vi "Orca Flash Engine.vi"(0 "Notifier Name":string, 11 "Camera ID":string[](array[string])) -> ()   [LabVIEW 2025]
uses:
  Orca Flash Controls/Orca Flash Parameters.ctl
  Orca Flash Controls/Orca Flash Parameter List.ctl
  Orca Flash Controls/Orca Flash ROI.ctl
  Orca Flash Controls/Orca Flash Notifier Element.ctl
  Orca Flash Controls/Orca Flash Actions.ctl
  <vilib>/vision/Image Controls.llb/IMAQ Image.ctl
  Camera Controls/Camera IMAQ Key Info.ctl
panel:
  out "Last Error":errorcluster
  in  "Ext Options":cluster{"Polarity":i32, "Delay":dbl}={"Polarity"=1, "Delay"=0.0} {"Polarity" items=["Negative"=1, "Positive"=2]}
  in  "Trigger Source":i32(ring)=1 items=["Internal"=1, "External"=2, "Software"=3, "Master Pulse"=4]
  in  "Port":i32=1
  in  "Options":cluster{"Width":dbl, "Delay":dbl, "Source":u32}={"Width"=0.003, "Delay"=0.0, "Source"=2} {"Source" items=["Exposure"=1, "Readout End"=2, "V Sync"=3, "H Sync"=4, "Trigger"=6]}
  in  "Trigger Type":cluster{"Mode":u32, "Polarity":u32}={"Mode"=1, "Polarity"=2} {"Mode" items=["Low"=1, "Global Exposure"=2, "Programmable"=3, "Trigger Ready"=4, "High"=5]; "Polarity" items=["Negative"=1, "Positive"=2]}
  in  "Orca Flash ROI":T1
  in  "Use Display Module":bool
  in  "Sensor Mode":enum32{"Area", "Progressive"}(radio)
  in  "Number of lines":dbl=8.0
  in  "Internal Line Interval Setpoint":dbl=0.001
  in  "Get Parameter":bool
  in  "Set Parameter":bool
  in  "Get ROI":bool
  in  "Set ROI":bool
  in  "sCMOS Parameter":T2={"Value"=0.0, "Parameter"=2049184} {"Parameter" items=["SENSOR MODE"=4212128, "READOUT SPEED"=4211872, "READOUT DIRECTION"=4211904, "TRIGGER GLOBAL EXPOSURE"=2049680, "TRIGGER DELAY"=1066480, "SYNC READOUT SYSTEM BLANK"=1066528, "SENSOR COOLER"=2115248, "SENSOR COOLER STATUS"=2115280, "EXPOSURE TIME"=2049184, "DEFECT CORRECT MODE"=4670368, "BINNING"=4215968, "INTERNAL LINE SPEED"=4226000, "INTERNAL LINE INTERVAL"=4226016, "IMAGE PIXEL TYPE"=4343296, "NUMBER OF OUTPUT TRIGGER CONNECTOR"=1852320, "OUTPUT TRIGGER SOURCE[0]"=1852576, "OUTPUT TRIGGER SOURCE[1]"=1852832, "OUTPUT TRIGGER SOURCE[2]"=1853088, "OUTPUT TRIGGER POLARITY[0]"=1852592, "OUTPUT TRIGGER POLARITY[1]"=1852848, "OUTPUT TRIGGER POLARITY[2]"=1853104, "OUTPUT TRIGGER ACTIVE[0]"=1852608, "OUTPUT TRIGGER ACTIVE[1]"=1852864, "OUTPUT TRIGGER ACTIVE[2]"=1853120, "OUTPUT TRIGGER DELAY[0]"=1852624, "OUTPUT TRIGGER DELAY[1]"=1852880, "OUTPUT TRIGGER DELAY[2]"=1853136, "OUTPUT TRIGGER PERIOD[0]"=1852640, "OUTPUT TRIGGER PERIOD[1]"=1852896, "OUTPUT TRIGGER PERIOD[2]"=1853152, "OUTPUT TRIGGER KIND[0]"=1852656, "OUTPUT TRIGGER KIND[1]"=1852912, "OUTPUT TRIGGER KIND[2]"=1853168, "OUTPUT TRIGGER PRE HSYNC COUNT"=1852704]}
  in  "# of frames":u32=100
  in  "Path":path
  in  "Record":bool
  in  "Preview":bool
  out "Acquisition Loop":i32
  in  "QUIT":bool
  out "Acquisition Frame":i32
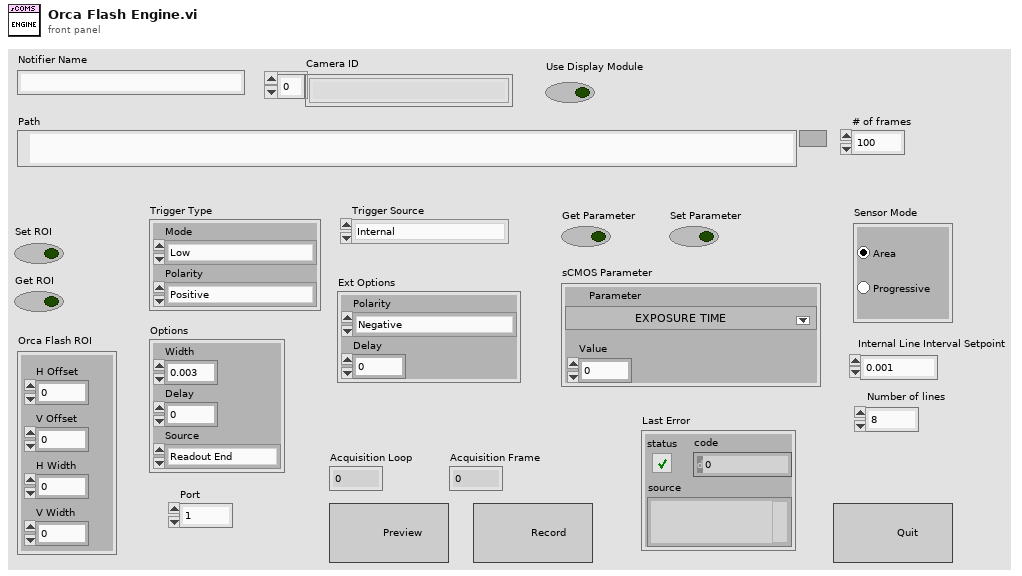
[diagram p1: front panel]
types:
  T1 = typedef "Orca Flash ROI.ctl" = cluster{"H Offset":i32, "V Offset":i32, "H Width":i32, "V Width":i32}
  T2 = typedef "Orca Flash Parameters.ctl" = cluster{"Value":dbl, "Parameter":T3}
  T3 = typedef "Orca Flash Parameter List.ctl" = u32
  T4 = typedef "Camera IMAQ Key Info.ctl" = cluster{"Frame":u32, "Sensor Height":i32, "Sensor Width":i32, "ROI Height":i32, "ROI Width":i32, "ROI Enable?":bool, "Bit per Pixel":u8}
  T5 = typedef "Image Type" = u32
  T6 = typedef "Orca Flash Notifier Element.ctl" = cluster{"Camera Actions":T7, "Received?":bool, "Running?":bool, "sCMOS Parameter":T2, "sCMOS ROI":T1, "Save Path":path, "# of frames":u32, "Image Ref":T8}
  T7 = typedef "Orca Flash Actions.ctl" = enum16{"Idle", "Preview", "Record", "Record Settings", "Set Param", "Get Param", "Set ROI", "Get ROI", "Trigger Source", "Trigger Type", "Progessive Mode", "Area Mode", "Status", "Quit"}
  T8 = typedef "IMAQ Image.ctl" = refnum<image>
  T9 = enum32{"Invalid", "Standard", "Closed", "Hidden", "Minimized", "Maximized"}
  T10 = cluster{"Horizontal Offset":i32, "Vertical Offset":i32, "Horizontal Size":i32, "Vertical Size":i32}
  T11 = typedef "LVMinMaxIncTypeDef.ctl" = cluster{"Minimum":dbl, "Maximum":dbl, "Increment":dbl}
  T12 = cluster{"H Offset":cluster{"Value":i32, "Limits":T11}, "V Offset":cluster{"Value":i32, "Limits":T11}, "H Size":cluster{"Value":i32, "Limits":T11}, "V Size":cluster{"Value":i32, "Limits":T11}}
  T13 = cluster{"Input Trigger Mode":u32, "Input Trigger Polarity":u32, "Times":u32, "Delay":dbl}
  T14 = cluster{"Output Trigger Period":dbl, "Delay":dbl, "Source":u32}
  T15 = cluster{"Output Trigger Mode":u32, "Output Trigger Polarity":u32}
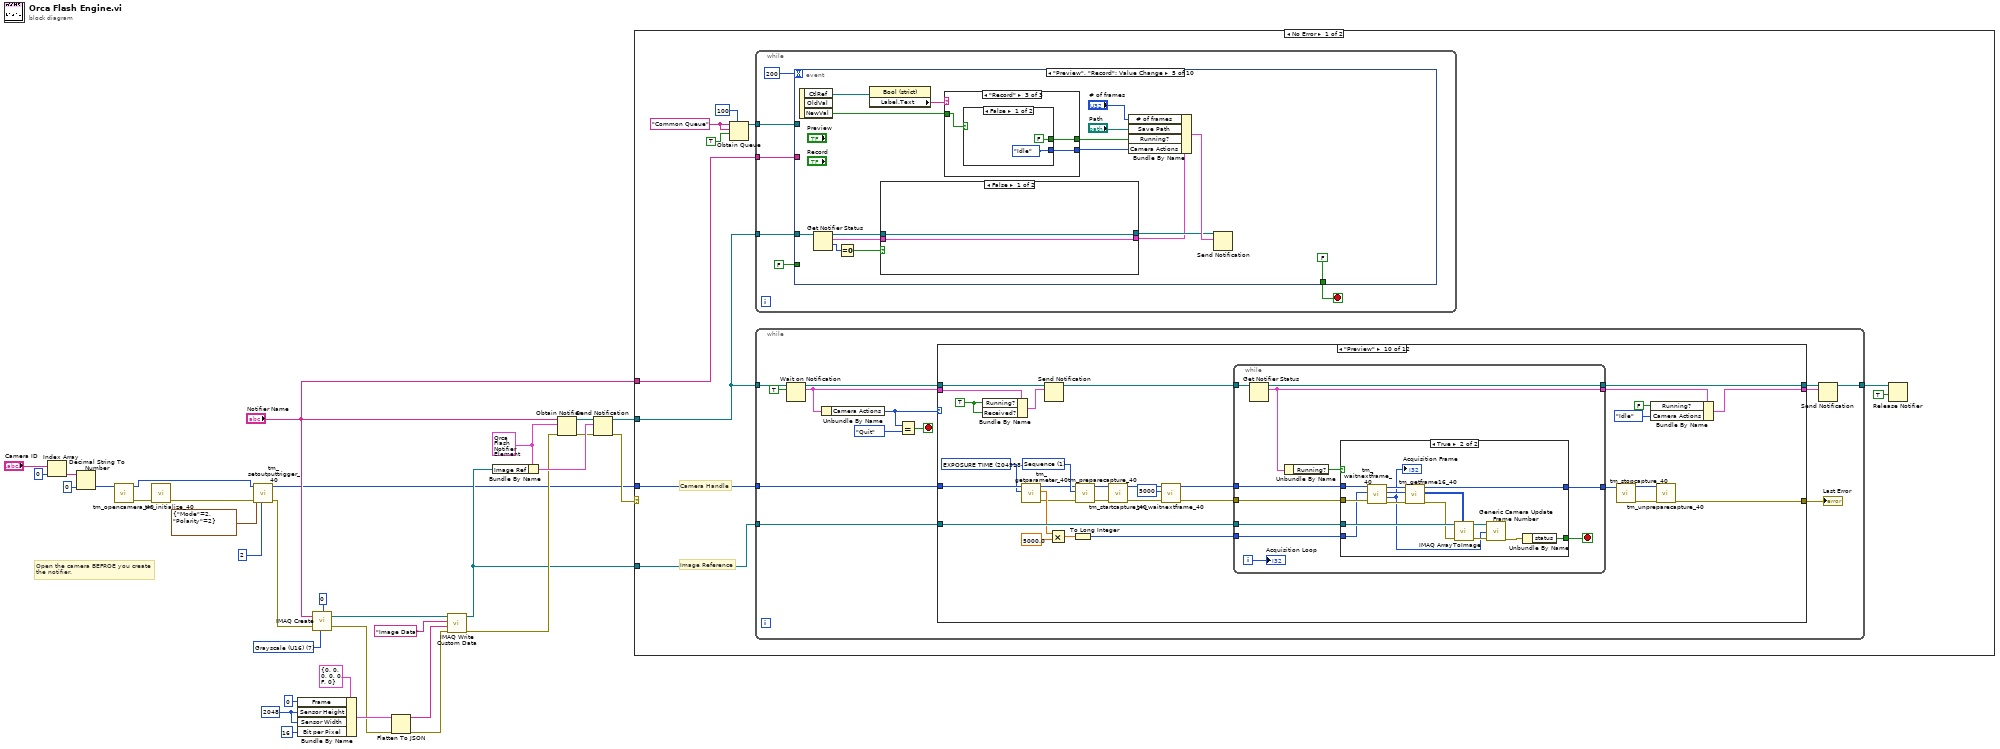
[diagram p0: block diagram]
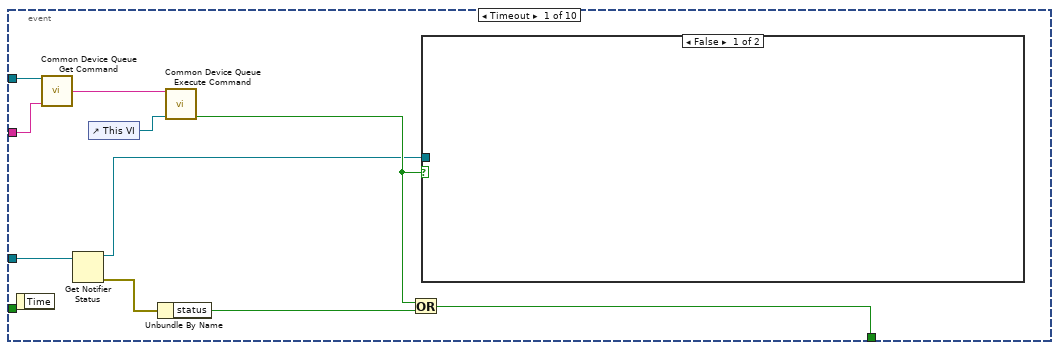
[diagram p2: hidden frame]
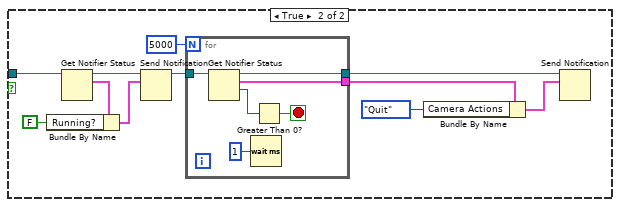
[diagram p3: hidden frame]
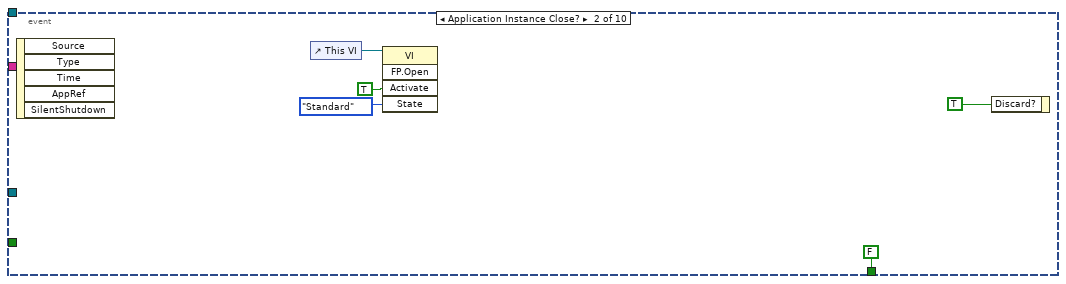
[diagram p4: hidden frame]
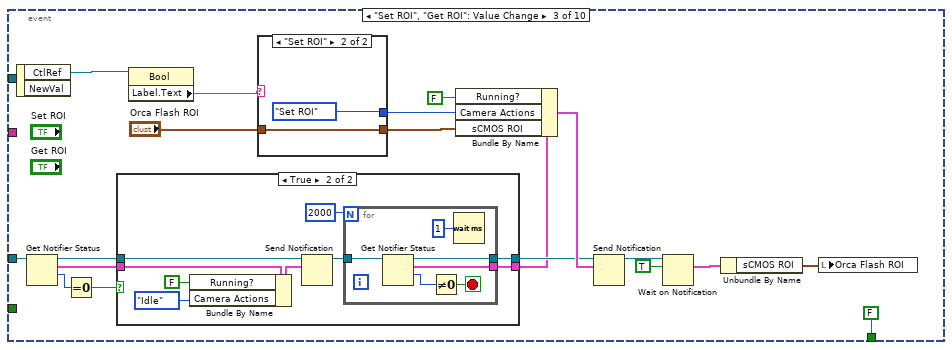
[diagram p5: hidden frame]
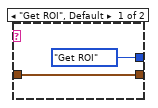
[diagram p7: hidden frame]
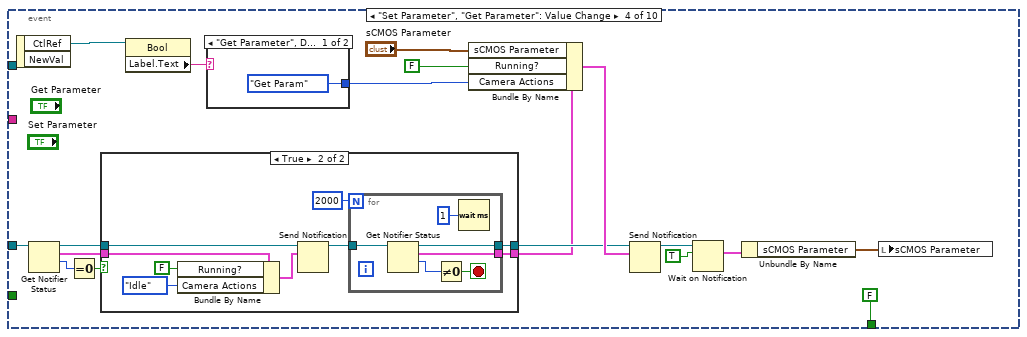
[diagram p8: hidden frame]
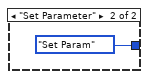
[diagram p10: hidden frame]
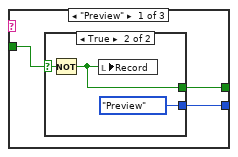
[diagram p11: hidden frame]
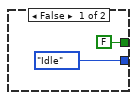
[diagram p12: hidden frame]
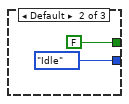
[diagram p13: hidden frame]
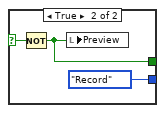
[diagram p14: hidden frame]
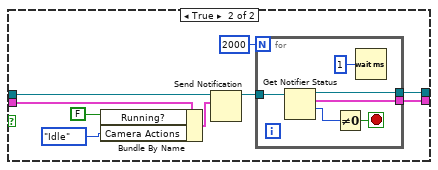
[diagram p15: hidden frame]
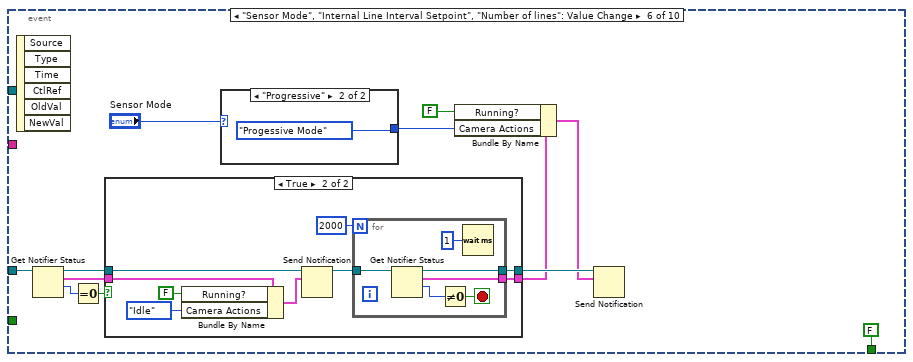
[diagram p16: hidden frame]
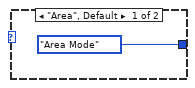
[diagram p17: hidden frame]
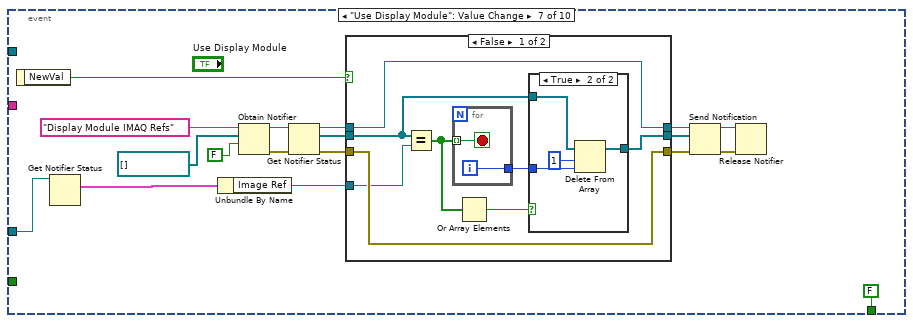
[diagram p19: hidden frame]
diagram:
  w18 = 2048 ("Sensor Height")
  w14 = T5 7 items=["Grayscale (U8)", "Grayscale (I16)", "Grayscale (SGL)", "Complex (CSG)", "RGB (U32)", "HSL (U32)", "RGB (U64)", "Grayscale (U16)"] ("Image Type")
  w28 = T6 {"Camera Actions"=enum."Idle", "Received?"=FALSE, "Running?"=FALSE, "sCMOS Parameter"={"Value"=0.0, "Parameter"=0}, "sCMOS ROI"={"H Offset"=0, "V Offset"=0, "H Width"=0, "V Width"=0}, "Save Path"=path "", "# of frames"=1, "Image Ref"=refnum} ("Camera Cluster")
  # "Open the camera BEFROE you create\nthe notifier."
  n1 = Index Array(array="Camera ID", index=0) -> (element=w31:string)
  n2 = Decimal String To Number(string=w31, default (0L)=u32 0 ("default (0 I32)")) -> (number=w24:u32)  [unwired: 1 in, 1 out]
  n3 = call <userlib>:"tm_initialize_40.vi"() -> ("error out"=w25:errorcluster)  [unwired: 8 in, 3 out]
  n4 = call <userlib>:"tm_opencamera_40.vi"("error in (no error)"=w25, "Camera Index"=w24) -> ("error out"=w4:errorcluster, "Handle out"=w3:u32)  [unwired: 7 in, 1 out]
  n5 = call <userlib>:"tm_setoutputtrigger_40.vi"("Port"=2, "error in (no error)"=w4, "Type"=cluster{"Mode":u32, "Polarity":u32} {"Mode"=2, "Polarity"=2}, "Handle in"=w3) -> ("error out"=w6:errorcluster, "Handle out"=w5:u32)  [unwired: 6 in]
  n6 = Bundle By Name(cluster=T4 {"Frame"=0, "Sensor Height"=0, "Sensor Width"=0, "ROI Height"=0, "ROI Width"=0, "ROI Enable?"=FALSE, "Bit per Pixel"=0} ("Camera IMAQ Key Info"), "Frame"=u32 0, "Sensor Height"=w18, "Sensor Width"=w18, "Bit per Pixel"=u8 16) -> (w21:T4)
  n7 = call "IMAQ Create"("Border Size"=0, "Image Name"="Notifier Name", "Image Type"=w14, "error in (no error)"=w6) -> ("New Image"=w16:T8, "error out"=w13:errorcluster)  [unwired: 1 in]
  n8 = Flatten To JSON(anything=w21, error in (no error)=w13) -> (JSON string=w22:string, 11:w12:errorcluster)  [unwired: 1 in]
  n9 = call "IMAQ Write Custom Data"("error in (no error)"=w12, "Custom Data In"=w22, "Key"="Image Data", "Image"=w16) -> ("error out"=w11:errorcluster, "Image Out"=w8:T8)  [unwired: 6 in]
  n10 = Bundle By Name(cluster=w28, "Image Ref"=w8) -> (w29:T6)
  n11 = Obtain Notifier(name (unnamed)="Notifier Name", notification data type=w28, error in (no error)=w11) -> (notifier out=w27:refnum<notifier>, error out=w26:errorcluster)  [unwired: 1 in, 1 out]
  n12 = Send Notification(notification=w29, notifier=w27, error in (no error)=w26) -> (notifier out=w10:refnum<notifier>, error out=w7:errorcluster)
  n13 = case shown="No Error" w7 {
    selector: w7 -> [_ w719]
    tunnel: w10 -> [w37 w712]
    tunnel: "Notifier Name" -> [w34 w709]
    tunnel: w8 -> [w39 _]
    tunnel: w5 -> [w38 _]
    frame No Error {
      w43 = "Common Queue" ("Unique Notifier Name")
      # "Image Reference"
      # "Camera Handle"
      n14 = Obtain Queue(max queue size (-1, unlimited)=100, name (unnamed)=w43, element data type=w43, create if not found? (T)=TRUE) -> (queue out=w40:refnum<queue>)  [unwired: 1 in, 2 out]
      n15 = while {
        tunnel: w37 -> [w47]
        tunnel: w40 -> [w46]
        tunnel: w34 -> [w45]
        stop <- w49 stop-if-true
        n16 = event shown="[4] \"Preview\", \"Record\": Value Change" {
          selector: _ -> [_ _ _ _ _ _ _ _ _ _]
          dyn-events: _ -> [_ _ _ _ _ _ _ _ _ _]
          timeout: 200 -> [_ _ _ _ _ _ _ _ _ _]
          tunnel: w47 -> [w59 _ w88 w126 w169 w217 w241 w280 w308 w341]
          tunnel: [w56 FALSE ("NewVal") FALSE ("NewVal") FALSE ("NewVal") FALSE ("NewVal") FALSE ("NewVal") FALSE ("NewVal") w289 w317 w345] -> w49
          tunnel: w46 -> [w53 _ _ _ _ _ _ _ _ _]
          tunnel: w45 -> [w52 _ _ _ _ _ _ _ _ _]
          tunnel: FALSE -> [_ _ _ _ _ _ _ w289 w317 _]
          event Timeout {
            n17 = event-data() -> ()  [unwired: 1 in, 1 out]
            n18 = call "Common Device Queue Get Command.vi"("Common Queue"=w53, "Notifier Name"=w52) -> ("Command"=w55:string)  [unwired: 12 in, 1 out]
            n19 = Get Notifier Status(notifier=w59) -> (notifier out=w50:refnum<notifier>, error out=w58:errorcluster)  [unwired: 1 in, 3 out]
            n20 = control-ref of="This VI"() -> (w54:refnum<vi>)
            n21 = Unbundle By Name(w58) -> ("status"=w57:bool)
            n22 = call "Common Device Queue Execute Command.vi"("Common Command"=w55, "VI Refnum"=w54) -> ("Quit?"=w51:bool)  [unwired: 12 in, 1 out]
            n23 = Or(x=w51, y=w57) -> (x .or. y?=w56:bool)
            n24 = case shown="False" w51 {
              tunnel: w50 -> [_ w70]
              frame False {
              }
              frame True {
                n25 = Get Notifier Status(notifier=w70) -> (notifier out=w67:refnum<notifier>, current notification=w69:T6)  [unwired: 1 in, 3 out]
                n26 = Bundle By Name(cluster=w69, "Running?"=FALSE) -> (w66:T6)
                n27 = Send Notification(notification=w66, notifier=w67) -> (notifier out=w64:refnum<notifier>)  [unwired: 1 in, 1 out]
                n28 = for {
                  N: 5000 -> [_]
                  tunnel: w64 -> [w75]
                  tunnel: [w73] -> w63
                  tunnel: [w71] -> w62
                  stop <- w74 stop-if-true
                  n29 = Get Notifier Status(notifier=w75) -> (notifier out=w73:refnum<notifier>, current notification=w71:T6, # waiting=w76:i32)  [unwired: 1 in, 2 out]
                  n30 = Wait (ms)(milliseconds to wait=u32 1) -> ()  [unwired: 1 out]
                  n31 = Greater Than 0?(x=w76) -> (x > 0?=w74:bool)
                }
                n32 = Bundle By Name(cluster=w62, "Camera Actions"=Orca_Flash_Actions."Quit") -> (w60:T6)
                n33 = Send Notification(notification=w60, notifier=w63) -> ()  [unwired: 1 in, 2 out]
              }
            }
          }
          event Application Instance Close? {
            n34 = event-data() -> ()  [unwired: 1 in, 5 out]
            n35 = control-ref of="This VI"() -> (w79:refnum<vi>)
            n36 = invoke class="VI" method="FP.Open"(reference=w79, "Activate"=TRUE ("Activate?"), "State"=T9."Standard") -> ()  [unwired: 2 in, 5 out]
            n37 = event-data("Discard?"=TRUE) -> ()  [unwired: 1 in, 1 out]
          }
          event "Set ROI", "Get ROI": Value Change {
            n38 = event-data() -> ("CtlRef"=w98:refnum<vi>)  [unwired: 1 in, 1 out]
            n39 = Get Notifier Status(notifier=w88) -> (notifier out=w86:refnum<notifier>, current notification=w85:T6, # waiting=w84:i32)  [unwired: 1 in, 2 out]
            n40 = Equal To 0?(x=w84) -> (x = 0?=w87:bool)
            n41 = case shown="True" w87 {
              tunnel: [w102 w108] -> w90
              tunnel: [w101 w107] -> w89
              tunnel: w86 -> [w102 w106]
              tunnel: w85 -> [w101 w103]
              frame False {
              }
              frame True {
                n42 = Bundle By Name(cluster=w103, "Running?"=FALSE, "Camera Actions"=Orca_Flash_Actions."Idle") -> (w110:T6)
                n43 = Send Notification(notification=w110, notifier=w106) -> (notifier out=w111:refnum<notifier>)  [unwired: 1 in, 1 out]
                n44 = for {
                  N: 2000 -> [_]
                  tunnel: w111 -> [w117]
                  tunnel: [w114] -> w108
                  tunnel: [w113] -> w107
                  stop <- w115 stop-if-true
                  n45 = Get Notifier Status(notifier=w117) -> (notifier out=w114:refnum<notifier>, current notification=w113:T6, # waiting=w116:i32)  [unwired: 1 in, 2 out]
                  n46 = Not Equal To 0?(x=w116) -> (x != 0?=w115:bool)
                  n47 = Wait (ms)(milliseconds to wait=u32 1) -> ()  [unwired: 1 out]
                }
              }
            }
            n48 = property class="Bool"(reference=w98) -> ("Label.Text"=w97:string)  [unwired: 1 in, 2 out]
            n49 = case shown="\"Set ROI\"" w97 {
              tunnel: [Orca_Flash_Actions."Get ROI" ("Camera Actions") Orca_Flash_Actions."Set ROI" ("Camera Actions")] -> w96
              tunnel: [w118 w120] -> w95
              tunnel: "Orca Flash ROI" -> [w118 w120]
              frame "Get ROI", Default {
              }
              frame "Set ROI" {
              }
            }
            n50 = Bundle By Name(cluster=w89, "Running?"=FALSE, "Camera Actions"=w96, "sCMOS ROI"=w95) -> (w94:T6)
            n51 = Send Notification(notification=w94, notifier=w90) -> (notifier out=w93:refnum<notifier>)  [unwired: 1 in, 1 out]
            n52 = Wait on Notification(notifier=w93, ignore previous (F)=TRUE) -> (notification=w92:T6)  [unwired: 2 in, 3 out]
            n53 = Unbundle By Name(w92) -> ("sCMOS ROI"=w82:T1)
            n54 = local write "Orca Flash ROI"(w82) -> ()
          }
          event "Set Parameter", "Get Parameter": Value Change {
            n55 = event-data() -> ("CtlRef"=w137:refnum<vi>)  [unwired: 1 in, 1 out]
            n56 = Get Notifier Status(notifier=w126) -> (notifier out=w124:refnum<notifier>, current notification=w123:T6, # waiting=w122:i32)  [unwired: 1 in, 2 out]
            n57 = Equal To 0?(x=w122) -> (x = 0?=w125:bool)
            n58 = case shown="True" w125 {
              tunnel: w124 -> [w141 w150]
              tunnel: w123 -> [w140 w149]
              tunnel: [w141 w145] -> w129
              tunnel: [w140 w144] -> w128
              frame False {
              }
              frame True {
                n59 = Bundle By Name(cluster=w149, "Running?"=FALSE, "Camera Actions"=Orca_Flash_Actions."Idle") -> (w147:T6)
                n60 = Send Notification(notification=w147, notifier=w150) -> (notifier out=w146:refnum<notifier>)  [unwired: 1 in, 1 out]
                n61 = for {
                  N: 2000 -> [_]
                  tunnel: w146 -> [w156]
                  tunnel: [w153] -> w145
                  tunnel: [w152] -> w144
                  stop <- w154 stop-if-true
                  n62 = Get Notifier Status(notifier=w156) -> (notifier out=w153:refnum<notifier>, current notification=w152:T6, # waiting=w155:i32)  [unwired: 1 in, 2 out]
                  n63 = Not Equal To 0?(x=w155) -> (x != 0?=w154:bool)
                  n64 = Wait (ms)(milliseconds to wait=u32 1) -> ()  [unwired: 1 out]
                }
              }
            }
            n65 = property class="Bool"(reference=w137) -> ("Label.Text"=w136:string)  [unwired: 1 in, 2 out]
            n66 = case shown="\"Get Parameter\", Default" w136 {
              tunnel: [Orca_Flash_Actions."Get Param" ("Camera Actions") Orca_Flash_Actions."Set Param" ("Camera Actions")] -> w135
              frame "Get Parameter", Default {
              }
              frame "Set Parameter" {
              }
            }
            n67 = Bundle By Name(cluster=w128, "sCMOS Parameter"="sCMOS Parameter", "Running?"=FALSE, "Camera Actions"=w135) -> (w134:T6)
            n68 = Send Notification(notification=w134, notifier=w129) -> (notifier out=w133:refnum<notifier>)  [unwired: 1 in, 1 out]
            n69 = Wait on Notification(notifier=w133, ignore previous (F)=TRUE) -> (notification=w132:T6)  [unwired: 2 in, 3 out]
            n70 = Unbundle By Name(w132) -> ("sCMOS Parameter"=w131:T2)
            n71 = local write "sCMOS Parameter"(w131) -> ()
          }
          event "Preview", "Record": Value Change {
            n72 = event-data() -> ("CtlRef"=w173:refnum<vi>, "NewVal"=w171:bool)  [unwired: 1 in, 1 out]
            n73 = Get Notifier Status(notifier=w169) -> (notifier out=w161:refnum<notifier>, current notification=w160:T6, # waiting=w159:i32)  [unwired: 1 in, 2 out]
            n74 = Equal To 0?(x=w159) -> (x = 0?=w162:bool)
            n75 = property class="Bool (strict)"(reference=w173) -> ("Label.Text"=w172:string)  [unwired: 1 in, 2 out]
            n76 = case shown="False" w162 {
              tunnel: w161 -> [w194 w203]
              tunnel: [w194 w199] -> w164
              tunnel: [w193 w197] -> w163
              tunnel: w160 -> [w193 w196]
              frame False {
              }
              frame True {
                n77 = Bundle By Name(cluster=w196, "Running?"=FALSE, "Camera Actions"=Orca_Flash_Actions."Idle") -> (w201:T6)
                n78 = Send Notification(notification=w201, notifier=w203) -> (notifier out=w200:refnum<notifier>)  [unwired: 1 in, 1 out]
                n79 = for {
                  N: 2000 -> [_]
                  tunnel: w200 -> [w209]
                  tunnel: [w208] -> w199
                  tunnel: [w207] -> w197
                  stop <- w205 stop-if-true
                  n80 = Get Notifier Status(notifier=w209) -> (notifier out=w208:refnum<notifier>, current notification=w207:T6, # waiting=w206:i32)  [unwired: 1 in, 2 out]
                  n81 = Not Equal To 0?(x=w206) -> (x != 0?=w205:bool)
                  n82 = Wait (ms)(milliseconds to wait=u32 1) -> ()  [unwired: 1 out]
                }
              }
            }
            n83 = case shown="\"Record\"" w172 {
              tunnel: w171 -> [w177 _ w187]
              tunnel: [w176 FALSE w186] -> w167
              tunnel: [w175 Orca_Flash_Actions."Idle" ("Camera Actions") w185] -> w170
              frame "Preview" {
                n84 = case shown="True" w177 {
                  selector: w177 -> [_ w182]
                  tunnel: [FALSE w181] -> w176
                  tunnel: [Orca_Flash_Actions."Idle" ("Camera Actions") Orca_Flash_Actions."Preview" ("Camera Actions")] -> w175
                  frame False {
                  }
                  frame True {
                    n85 = Not(x=w182) -> (.not. x?=w181:bool)
                    n86 = local write "Record"(w181) -> ()
                  }
                }
              }
              frame Default {
              }
              frame "Record" {
                n87 = case shown="False" w187 {
                  selector: w187 -> [_ w192]
                  tunnel: [FALSE w191] -> w186
                  tunnel: [Orca_Flash_Actions."Idle" ("Camera Actions") Orca_Flash_Actions."Record" ("Camera Actions")] -> w185
                  frame False {
                  }
                  frame True {
                    n88 = Not(x=w192) -> (.not. x?=w191:bool)
                    n89 = local write "Preview"(w191) -> ()
                  }
                }
              }
            }
            n90 = Bundle By Name(cluster=w163, "# of frames"="# of frames", "Save Path"="Path", "Running?"=w167, "Camera Actions"=w170) -> (w168:T6)
            n91 = Send Notification(notification=w168, notifier=w164) -> ()  [unwired: 1 in, 2 out]
          }
          event "Sensor Mode", "Internal Line Interval Setpoint", "Number of lines": Value Change {
            n92 = event-data() -> ()  [unwired: 1 in, 6 out]
            n93 = Get Notifier Status(notifier=w217) -> (notifier out=w220:refnum<notifier>, current notification=w219:T6, # waiting=w218:i32)  [unwired: 1 in, 2 out]
            n94 = Equal To 0?(x=w218) -> (x = 0?=w221:bool)
            n95 = case shown="True" w221 {
              tunnel: w220 -> [w225 w234]
              tunnel: w219 -> [w224 w233]
              tunnel: [w225 w229] -> w216
              tunnel: [w224 w228] -> w215
              frame False {
              }
              frame True {
                n96 = Bundle By Name(cluster=w233, "Running?"=FALSE, "Camera Actions"=Orca_Flash_Actions."Idle") -> (w231:T6)
                n97 = Send Notification(notification=w231, notifier=w234) -> (notifier out=w230:refnum<notifier>)  [unwired: 1 in, 1 out]
                n98 = for {
                  N: 2000 -> [_]
                  tunnel: w230 -> [w240]
                  tunnel: [w237] -> w229
                  tunnel: [w236] -> w228
                  stop <- w238 stop-if-true
                  n99 = Get Notifier Status(notifier=w240) -> (notifier out=w237:refnum<notifier>, current notification=w236:T6, # waiting=w239:i32)  [unwired: 1 in, 2 out]
                  n100 = Not Equal To 0?(x=w239) -> (x != 0?=w238:bool)
                  n101 = Wait (ms)(milliseconds to wait=u32 1) -> ()  [unwired: 1 out]
                }
              }
            }
            n102 = case shown="\"Progressive\"" "Sensor Mode" {
              tunnel: [Orca_Flash_Actions."Area Mode" ("Camera Actions") Orca_Flash_Actions."Progessive Mode" ("Camera Actions")] -> w211
              frame "Area", Default {
              }
              frame "Progressive" {
              }
            }
            n103 = Bundle By Name(cluster=w215, "Running?"=FALSE, "Camera Actions"=w211) -> (w210:T6)
            n104 = Send Notification(notification=w210, notifier=w216) -> ()  [unwired: 1 in, 2 out]
          }
          event "Use Display Module": Value Change {
            n105 = event-data() -> ("NewVal"=w242:bool)  [unwired: 1 in]
            n106 = Get Notifier Status(notifier=w241) -> (current notification=w243:T6)  [unwired: 1 in, 4 out]
            n107 = Unbundle By Name(w243) -> ("Image Ref"=w257:T8)
            n108 = Obtain Notifier(name (unnamed)="Display Module IMAQ Refs", notification data type=T8[] [], create if not found? (T)=FALSE) -> (notifier out=w250:refnum<notifier>, error out=w251:errorcluster)  [unwired: 1 in, 1 out]
            n109 = Get Notifier Status(notifier=w250, error in (no error)=w251) -> (notifier out=w249:refnum<notifier>, current notification=w247:T8[], error out=w248:errorcluster)  [unwired: 2 out]
            n110 = case shown="False" w242 {
              tunnel: w249 -> [w266 w276]
              tunnel: w248 -> [w260 w275]
              tunnel: w247 -> [w262 w278]
              tunnel: [w261 w277] -> w244
              tunnel: [w266 w276] -> w246
              tunnel: [w260 w275] -> w245
              tunnel: w257 -> [w259 w274]
              frame False {
                n111 = Equal?(x=w262, y=w259) -> (x = y?=w265:bool[])
                n112 = for {
                  tunnel: w265 -> [w273] mode=indexing
                  tunnel: [w272] -> w263
                  i -> [w272]
                  stop <- w273 stop-if-true
                }
                n113 = Or Array Elements(Boolean array=w265) -> (logical OR=w264:bool)
                n114 = case shown="True" w264 {
                  tunnel: w263 -> [_ w270]
                  tunnel: w262 -> [w267 w269]
                  tunnel: [w267 w268] -> w261
                  frame False {
                  }
                  frame True {
                    n115 = Delete From Array(array=w269, length=1, index=w270) -> (array with subset deleted=w268:T8[])  [unwired: 1 out]
                  }
                }
              }
              frame True {
                n116 = Build Array (concatenate)(w278, w274) -> (w277:T8[])
              }
            }
            n117 = Send Notification(notification=w244, notifier=w246, error in (no error)=w245) -> (notifier out=w252:refnum<notifier>, error out=w253:errorcluster)
            n118 = Release Notifier(notifier=w252, error in (no error)=w253) -> ()  [unwired: 1 in, 3 out]
          }
          event "Trigger Type", "Options", "Port": Value Change {
            n119 = event-data() -> ()  [unwired: 1 in, 1 out]
            n120 = Get Notifier Status(notifier=w280) -> (notifier out=w287:refnum<notifier>, current notification=w286:T6, # waiting=w285:i32)  [unwired: 1 in, 2 out]
            n121 = Equal To 0?(x=w285) -> (x = 0?=w288:bool)
            n122 = case shown="True" w288 {
              tunnel: w287 -> [w291 w300]
              tunnel: w286 -> [w290 w299]
              tunnel: [w291 w295] -> w284
              tunnel: [w290 w294] -> w283
              frame False {
              }
              frame True {
                n123 = Bundle By Name(cluster=w299, "Running?"=FALSE, "Camera Actions"=Orca_Flash_Actions."Idle") -> (w297:T6)
                n124 = Send Notification(notification=w297, notifier=w300) -> (notifier out=w296:refnum<notifier>)  [unwired: 1 in, 1 out]
                n125 = for {
                  N: 2000 -> [_]
                  tunnel: w296 -> [w306]
                  tunnel: [w303] -> w295
                  tunnel: [w302] -> w294
                  stop <- w304 stop-if-true
                  n126 = Get Notifier Status(notifier=w306) -> (notifier out=w303:refnum<notifier>, current notification=w302:T6, # waiting=w305:i32)  [unwired: 1 in, 2 out]
                  n127 = Not Equal To 0?(x=w305) -> (x != 0?=w304:bool)
                  n128 = Wait (ms)(milliseconds to wait=u32 1) -> ()  [unwired: 1 out]
                }
              }
            }
            n129 = Bundle By Name(cluster=w283, "Running?"=FALSE, "Camera Actions"=Orca_Flash_Actions."Trigger Type") -> (w281:T6)
            n130 = Send Notification(notification=w281, notifier=w284) -> ()  [unwired: 1 in, 2 out]
          }
          event "Trigger Source", "Ext Options": Value Change {
            n131 = event-data() -> ()  [unwired: 1 in, 1 out]
            n132 = Get Notifier Status(notifier=w308) -> (notifier out=w315:refnum<notifier>, current notification=w314:T6, # waiting=w313:i32)  [unwired: 1 in, 2 out]
            n133 = Equal To 0?(x=w313) -> (x = 0?=w316:bool)
            n134 = case shown="True" w316 {
              tunnel: w315 -> [w319 w328]
              tunnel: w314 -> [w318 w327]
              tunnel: [w319 w323] -> w312
              tunnel: [w318 w322] -> w311
              frame False {
              }
              frame True {
                n135 = Bundle By Name(cluster=w327, "Running?"=FALSE, "Camera Actions"=Orca_Flash_Actions."Idle") -> (w325:T6)
                n136 = Send Notification(notification=w325, notifier=w328) -> (notifier out=w324:refnum<notifier>)  [unwired: 1 in, 1 out]
                n137 = for {
                  N: 2000 -> [_]
                  tunnel: w324 -> [w334]
                  tunnel: [w331] -> w323
                  tunnel: [w330] -> w322
                  stop <- w332 stop-if-true
                  n138 = Get Notifier Status(notifier=w334) -> (notifier out=w331:refnum<notifier>, current notification=w330:T6, # waiting=w333:i32)  [unwired: 1 in, 2 out]
                  n139 = Not Equal To 0?(x=w333) -> (x != 0?=w332:bool)
                  n140 = Wait (ms)(milliseconds to wait=u32 1) -> ()  [unwired: 1 out]
                }
              }
            }
            n141 = Bundle By Name(cluster=w311, "Running?"=FALSE, "Camera Actions"=Orca_Flash_Actions."Trigger Source") -> (w309:T6)
            n142 = Send Notification(notification=w309, notifier=w312) -> ()  [unwired: 1 in, 2 out]
          }
          event "QUIT": Value Change {
            n143 = event-data() -> ("NewVal"=w345:bool)  [unwired: 1 in]
            n144 = Get Notifier Status(notifier=w341) -> (notifier out=w337:refnum<notifier>, current notification=w336:T6, # waiting=w335:i32)  [unwired: 1 in, 2 out]
            n145 = Equal To 0?(x=w335) -> (x = 0?=w338:bool)
            n146 = case shown="True" w338 {
              tunnel: w337 -> [w347 w352]
              tunnel: [w347 w350] -> w340
              tunnel: [w346 w349] -> w339
              tunnel: w336 -> [w346 w348]
              frame False {
              }
              frame True {
                n147 = Bundle By Name(cluster=w348, "Running?"=FALSE, "Camera Actions"=Orca_Flash_Actions."Idle") -> (w351:T6)
                n148 = Send Notification(notification=w351, notifier=w352) -> (notifier out=w355:refnum<notifier>)  [unwired: 1 in, 1 out]
                n149 = for {
                  N: 2000 -> [_]
                  tunnel: w355 -> [w362]
                  tunnel: [w359] -> w350
                  tunnel: [w358] -> w349
                  stop <- w360 stop-if-true
                  n150 = Get Notifier Status(notifier=w362) -> (notifier out=w359:refnum<notifier>, current notification=w358:T6, # waiting=w361:i32)  [unwired: 1 in, 2 out]
                  n151 = Not Equal To 0?(x=w361) -> (x != 0?=w360:bool)
                  n152 = Wait (ms)(milliseconds to wait=u32 1) -> ()  [unwired: 1 out]
                }
              }
            }
            n153 = Bundle By Name(cluster=w339, "Running?"=FALSE, "Camera Actions"=Orca_Flash_Actions."Quit") -> (w344:T6)
            n154 = Send Notification(notification=w344, notifier=w340) -> ()  [unwired: 1 in, 2 out]
          }
        }
      }
      n155 = while {
        tunnel: w37 -> [w375]
        tunnel: w39 -> [w374]
        tunnel: w38 -> [w373]
        tunnel: [w372] -> w35
        stop <- w371 stop-if-true
        n156 = Wait on Notification(notifier=w375, ignore previous (F)=TRUE) -> (notifier out=w368:refnum<notifier>, notification=w367:T6)  [unwired: 2 in, 2 out]
        n157 = Unbundle By Name(w367) -> ("Camera Actions"=w365:T7)
        n158 = Equal?(x=w365, y=Orca_Flash_Actions."Quit") -> (x = y?=w371:bool)
        n159 = case shown="\"Preview\"" w365 {
          tunnel: w373 -> [_ w386 w430 w433 w478 w487 w502 w534 w559 w581 w637 w702]
          tunnel: [errorcluster {"status"=FALSE, "code"=0, "source"=""} ("error out") w384 w429 w462 w477 w486 w501 w522 w549 w589 w649 w701] -> w363
          tunnel: w368 -> [w380 w390 w431 w469 w483 w485 w500 w548 w568 w599 w667 w708]
          tunnel: w374 -> [_ _ _ w444 _ _ _ _ _ w586 w646 w703]
          tunnel: w367 -> [w378 w382 w427 w465 w480 w484 w499 w545 w556 w594 w658 w706]
          tunnel: [w380 w390 w431 w469 w483 w485 w500 w548 w568 w595 w659 w708] -> w369
          tunnel: [w377 w389 w423 w464 w479 w484 w499 w544 w555 w590 w654 w705] -> w366
          frame "Idle", Default {
            w379 = FALSE ("Running?")
            n160 = Bundle By Name(cluster=w378, "Received?"=w379, "Running?"=w379) -> (w377:T6)
          }
          frame "Set Param" {
            n161 = Unbundle By Name(w382) -> ("sCMOS Parameter.Parameter"=w381:T3, "sCMOS Parameter.Value"=w385:dbl)
            n162 = case shown="Default" w381 {
              selector: w381 -> [w392 _]
              tunnel: w386 -> [w399 w405]
              tunnel: w385 -> [w398 w415]
              tunnel: [w396 w406] -> w384
              tunnel: [w394 0.0 ("Value out")] -> w383
              frame Default {
                w393 = u32 4212128 items=["SENSOR MODE"=4212128, "READOUT SPEED"=4211872, "READOUT DIRECTION"=4211904, "TRIGGER GLOBAL EXPOSURE"=2049680, "TRIGGER DELAY"=1066480, "INTERNAL TRIGGER HANDLING"=1066496, "SYNC READOUT SYSTEM BLANK"=1066528, "SENSOR TEMPERATURE"=2115232, "SENSOR COOLER STATUS"=2115280, "EXPOSURE TIME"=2049184, "DEFECT CORRECT MODE"=4670368, "BINNING"=4215968, "INTERNAL LINE SPEED"=4226000, "INTERNAL LINE INTERVAL"=4226016, "NUMBER OF OUTPUT TRIGGER CONNECTOR"=1852320, "OUTPUT TRIGGER SOURCE[0]"=1852576, "OUTPUT TRIGGER SOURCE[1]"=1852832, "OUTPUT TRIGGER SOURCE[2]"=1853088, "OUTPUT TRIGGER POLARITY[0]"=1852592, "OUTPUT TRIGGER POLARITY[1]"=1852848, "OUTPUT TRIGGER POLARITY[2]"=1853104, "OUTPUT TRIGGER ACTIVE[0]"=1852608, "OUTPUT TRIGGER ACTIVE[1]"=1852864, "OUTPUT TRIGGER ACTIVE[2]"=1853120, "OUTPUT TRIGGER DELAY[0]"=1852624, "OUTPUT TRIGGER DELAY[1]"=1852880, "OUTPUT TRIGGER DELAY[2]"=1853136, "OUTPUT TRIGGER PERIOD[0]"=1852640, "OUTPUT TRIGGER PERIOD[1]"=1852896, "OUTPUT TRIGGER PERIOD[2]"=1853152, "OUTPUT TRIGGER KIND[0]"=1852656, "OUTPUT TRIGGER KIND[1]"=1852912, "OUTPUT TRIGGER KIND[2]"=1853168, "OUTPUT TRIGGER BASE SENSOR[0]"=1852672, "OUTPUT TRIGGER BASE SENSOR[1]"=1852928, "OUTPUT TRIGGER BASE SENSOR[2]"=1853184, "OUTPUT TRIGGER PRE HSYNC COUNT"=1852704] ("Parameter")
                n163 = Type Cast(type=w393, x=w392) -> (*(type *) &x=w391:u32)
                n164 = call <userlib>:"tm_setparameter_40.vi"("Value in"=w398, "Parameter"=w391, "Handle in"=w399) -> ("error out"=w397:errorcluster, "Handle out"=w395:u32)  [unwired: 7 in]
                n165 = call <userlib>:"tm_getparameter_40.vi"("error in (no error)"=w397, "Parameter"=w391, "Handle in"=w395) -> ("error out"=w396:errorcluster, "Value out"=w394:dbl)  [unwired: 6 in, 1 out]
              }
              frame 0 {
                w401 = 1 items=["Internal"=1, "External"=2, "Software"=3, "Master Pulse"=4] ("Trigger Source 2")
                w403 = 2 items=["Internal"=1, "External"=2, "Software"=3, "Master Pulse"=4] ("Trigger Source 2")
                n166 = Greater Than 0?(x=w415) -> (x > 0?=w404:bool)
                n167 = Select(t=w403, s=w404, f=w401) -> (s? t:f=w402:i32)
                n168 = call <userlib>:"tm_inputtriggersource_40.vi"("External Options"=cluster{"Polarity":i32, "Delay":dbl} {"Polarity"=2, "Delay"=0.0} ("Ext Options 2"), "Source"=w402, "Handle in"=w405) -> ("error out"=w412:errorcluster, "Handle out"=w411:u32)  [unwired: 7 in]
                n169 = case shown="2" w402 {
                  tunnel: w411 -> [w417 w422]
                  tunnel: w412 -> [w416 w421]
                  tunnel: [w417 w419] -> w413
                  tunnel: [w416 w418] -> w414
                  frame Default {
                  }
                  frame 2 {
                    w420 = 1 items=["Edge"=1, "Level"=2, "Sync Readout"=3, "Point"=4] ("Active")
                    n170 = call <userlib>:"tm_inputtriggeractive_40.vi"("error in (no error)"=w421, "Active"=w420, "Handle in"=w422) -> ("error out"=w418:errorcluster, "Handle out"=w419:u32)  [unwired: 7 in]
                  }
                }
                n171 = call <userlib>:"tm_setoutputtrigger_40.vi"("Port"=0 ("Port 2"), "error in (no error)"=w414, "Programmable Options"=cluster{"Width":dbl, "Delay":dbl, "Source":u32} {"Width"=0.003, "Delay"=0.0, "Source"=2} ("Options 2"), "Type"=cluster{"Mode":u32, "Polarity":u32} {"Mode"=4, "Polarity"=2} ("Trigger Type 2"), "Handle in"=w413) -> ("error out"=w406:errorcluster)  [unwired: 5 in, 1 out]
              }
            }
            n172 = Bundle By Name(cluster=w382, "Received?"=TRUE ("Running?"), "Camera Actions"=Orca_Flash_Actions."Idle", "sCMOS Parameter.Value"=w383) -> (w389:T6)
          }
          frame "Get Param" {
            n173 = Unbundle By Name(w427) -> ("sCMOS Parameter.Parameter"=w428:T3)
            n174 = call <userlib>:"tm_getparameter_40.vi"("Parameter"=w428, "Handle in"=w430) -> ("error out"=w429:errorcluster, "Value out"=w424:dbl)  [unwired: 7 in, 1 out]
            n175 = Bundle By Name(cluster=w427, "Received?"=TRUE ("Running?"), "Camera Actions"=Orca_Flash_Actions."Idle", "sCMOS Parameter.Value"=w424) -> (w423:T6)
          }
          frame "Set ROI" {
            w451 = "Image Data" ("Key")
            n176 = Unbundle By Name(w465) -> ("sCMOS ROI.H Offset"=w441:i32, "sCMOS ROI.V Offset"=w440:i32, "sCMOS ROI.H Width"=w439:i32, "sCMOS ROI.V Width"=w438:i32)
            n177 = call "Orca Flash Fix ROI Size.vi"("Requested Value 1"=w441, "Allowed Increment"=4, "Requested Value 2"=w440, "Requested Value 3"=w439, "Requested Value 4"=w438) -> ("Resulting Value 1"=w437:i32, "Resulting Value 2"=w436:i32, "Resulting Value 3"=w435:i32, "Resulting Value 4"=w434:i32)  [unwired: 7 in]
            n178 = Bundle By Name(cluster=T10 {"Horizontal Offset"=0, "Vertical Offset"=0, "Horizontal Size"=0, "Vertical Size"=0} ("Sub Region"), "Horizontal Offset"=w437, "Vertical Offset"=w436, "Horizontal Size"=w435, "Vertical Size"=w434) -> (w455:T10)
            n179 = call <userlib>:"tm_setarea_40.vi"("Sub Region"=w455, "Handle in"=w433) -> ("error out"=w463:errorcluster, "Handle out"=w468:u32)  [unwired: 8 in]
            n180 = call <userlib>:"tm_getarea_40.vi"("error in (no error)"=w463, "Handle in"=w468) -> ("error out"=w462:errorcluster, "Sub Region"=w461:T12)  [unwired: 7 in, 1 out]
            n181 = Unbundle By Name(w461) -> ("H Offset.Value"=w459:i32, "V Offset.Value"=w458:i32, "H Size.Value"=w442:i32, "V Size.Value"=w443:i32)
            n182 = Bundle By Name(cluster=T1 {"H Offset"=0, "V Offset"=0, "H Width"=0, "V Width"=0} ("Orca Flash ROI"), "H Offset"=w459, "V Offset"=w458, "H Width"=w442, "V Width"=w443) -> (w457:T1)
            n183 = Bundle By Name(cluster=w465, "Received?"=TRUE ("Running?"), "Camera Actions"=Orca_Flash_Actions."Idle", "sCMOS ROI"=w457) -> (w464:T6)
            n184 = call "IMAQ Read Custom Data"("Key"=w451, "Image"=w444) -> ("error out"=w452:errorcluster, "Custom Data Out"=w447:string, "Image (duplicate)"=w445:T8)  [unwired: 7 in]
            n185 = Unflatten From JSON(JSON string=w447, type and defaults=T4 {"Frame"=0, "Sensor Height"=0, "Sensor Width"=0, "ROI Height"=0, "ROI Width"=0, "ROI Enable?"=FALSE, "Bit per Pixel"=0} ("Camera IMAQ Key Info"), error in (no error)=w452) -> (value=w448:T4, error out=w453:errorcluster)  [unwired: 4 in]
            n186 = Bundle By Name(cluster=w448, "ROI Width"=w442, "ROI Height"=w443) -> (w449:T4)
            n187 = Flatten To JSON(anything=w449, error in (no error)=w453) -> (JSON string=w450:string, 11:w454:errorcluster)  [unwired: 1 in]
            n188 = call "IMAQ Write Custom Data"("error in (no error)"=w454, "Custom Data In"=w450, "Key"=w451, "Image"=w445) -> ()  [unwired: 6 in, 2 out]
          }
          frame "Get ROI" {
            n189 = call <userlib>:"tm_getarea_40.vi"("Handle in"=w478) -> ("error out"=w477:errorcluster, "Sub Region"=w476:T12)  [unwired: 8 in, 1 out]
            n190 = Unbundle By Name(w476) -> ("H Offset.Value"=w471:i32, "V Offset.Value"=w472:i32, "H Size.Value"=w473:i32, "V Size.Value"=w474:i32)
            n191 = Bundle By Name(cluster=T1 {"H Offset"=0, "V Offset"=0, "H Width"=0, "V Width"=0} ("Orca Flash ROI"), "H Offset"=w471, "V Offset"=w472, "H Width"=w473, "V Width"=w474) -> (w470:T1)
            n192 = Bundle By Name(cluster=w480, "Received?"=TRUE ("Running?"), "Camera Actions"=Orca_Flash_Actions."Idle", "sCMOS ROI"=w470) -> (w479:T6)
          }
          frame "Trigger Source" {
            n193 = call <userlib>:"tm_inputtriggersource_40.vi"("External Options"="Ext Options", "Source"="Trigger Source", "Handle in"=w487) -> ("error out"=w490:errorcluster, "Handle out"=w489:u32)  [unwired: 7 in]
            n194 = case shown="2" "Trigger Source" {
              tunnel: w489 -> [w493 w498]
              tunnel: w490 -> [w492 w497]
              tunnel: [w493 w495] -> _
              tunnel: [w492 w494] -> w486
              frame Default {
              }
              frame 2 {
                w496 = 1 items=["Edge"=1, "Level"=2, "Sync Readout"=3, "Point"=4] ("Active")
                n195 = call <userlib>:"tm_inputtriggeractive_40.vi"("error in (no error)"=w497, "Active"=w496, "Handle in"=w498) -> ("error out"=w494:errorcluster, "Handle out"=w495:u32)  [unwired: 7 in]
              }
            }
          }
          frame "Trigger Type" {
            n196 = call <userlib>:"tm_setoutputtrigger_40.vi"("Port"="Port", "Programmable Options"="Options", "Type"="Trigger Type", "Handle in"=w502) -> ("error out"=w501:errorcluster)  [unwired: 6 in, 1 out]
          }
          frame "Progessive Mode" {
            w511 = u32 2 items=["Exposure"=1, "Readout End"=2, "V Sync"=3, "H Sync"=4, "Trigger"=6] ("Source")
            w513 = u32 2 items=["NEGATIVE"=1, "POSITIVE"=2] ("Output Trigger Polarity")
            w512 = u32 3 items=["LOW"=1, "GLOBAL EXPOSURE"=2, "PROGRAMMABLE"=3, "TRIGGER READY"=4, "HIGH"=5] ("Output Trigger Mode")
            w520 = u32 2 items=["NEGATIVE"=1, "POSITIVE"=2] ("Input Trigger Polarity")
            w519 = u32 1 items=["INTERNAL"=1, "EXTERNAL EDGE"=2, "EXTERNAL LEVEL"=4, "SOFTWARE"=32, "FAST REPETITION"=64, "TDI"=128, "START"=512, "SYNC READOUT"=1024] ("Input Trigger Mode")
            w521 = u32 2049184 items=["SENSOR MODE"=4212128, "READOUT SPEED"=4211872, "READOUT DIRECTION"=4211904, "TRIGGER GLOBAL EXPOSURE"=2049680, "TRIGGER DELAY"=1066480, "INTERNAL TRIGGER HANDLING"=1066496, "SYNC READOUT SYSTEM BLANK"=1066528, "SENSOR TEMPERATURE"=2115232, "SENSOR COOLER STATUS"=2115280, "EXPOSURE TIME"=2049184, "DEFECT CORRECT MODE"=4670368, "BINNING"=4215968, "INTERNAL LINE SPEED"=4226000, "INTERNAL LINE INTERVAL"=4226016, "NUMBER OF OUTPUT TRIGGER CONNECTOR"=1852320, "OUTPUT TRIGGER SOURCE[0]"=1852576, "OUTPUT TRIGGER SOURCE[1]"=1852832, "OUTPUT TRIGGER SOURCE[2]"=1853088, "OUTPUT TRIGGER POLARITY[0]"=1852592, "OUTPUT TRIGGER POLARITY[1]"=1852848, "OUTPUT TRIGGER POLARITY[2]"=1853104, "OUTPUT TRIGGER ACTIVE[0]"=1852608, "OUTPUT TRIGGER ACTIVE[1]"=1852864, "OUTPUT TRIGGER ACTIVE[2]"=1853120, "OUTPUT TRIGGER DELAY[0]"=1852624, "OUTPUT TRIGGER DELAY[1]"=1852880, "OUTPUT TRIGGER DELAY[2]"=1853136, "OUTPUT TRIGGER PERIOD[0]"=1852640, "OUTPUT TRIGGER PERIOD[1]"=1852896, "OUTPUT TRIGGER PERIOD[2]"=1853152, "OUTPUT TRIGGER KIND[0]"=1852656, "OUTPUT TRIGGER KIND[1]"=1852912, "OUTPUT TRIGGER KIND[2]"=1853168, "OUTPUT TRIGGER BASE SENSOR[0]"=1852672, "OUTPUT TRIGGER BASE SENSOR[1]"=1852928, "OUTPUT TRIGGER BASE SENSOR[2]"=1853184, "OUTPUT TRIGGER PRE HSYNC COUNT"=1852704] ("Parameter")
            w527 = u32 4226016 items=["SENSOR MODE"=4212128, "READOUT SPEED"=4211872, "READOUT DIRECTION"=4211904, "TRIGGER GLOBAL EXPOSURE"=2049680, "TRIGGER DELAY"=1066480, "INTERNAL TRIGGER HANDLING"=1066496, "SYNC READOUT SYSTEM BLANK"=1066528, "SENSOR TEMPERATURE"=2115232, "SENSOR COOLER STATUS"=2115280, "EXPOSURE TIME"=2049184, "DEFECT CORRECT MODE"=4670368, "BINNING"=4215968, "INTERNAL LINE SPEED"=4226000, "INTERNAL LINE INTERVAL"=4226016, "NUMBER OF OUTPUT TRIGGER CONNECTOR"=1852320, "OUTPUT TRIGGER SOURCE[0]"=1852576, "OUTPUT TRIGGER SOURCE[1]"=1852832, "OUTPUT TRIGGER SOURCE[2]"=1853088, "OUTPUT TRIGGER POLARITY[0]"=1852592, "OUTPUT TRIGGER POLARITY[1]"=1852848, "OUTPUT TRIGGER POLARITY[2]"=1853104, "OUTPUT TRIGGER ACTIVE[0]"=1852608, "OUTPUT TRIGGER ACTIVE[1]"=1852864, "OUTPUT TRIGGER ACTIVE[2]"=1853120, "OUTPUT TRIGGER DELAY[0]"=1852624, "OUTPUT TRIGGER DELAY[1]"=1852880, "OUTPUT TRIGGER DELAY[2]"=1853136, "OUTPUT TRIGGER PERIOD[0]"=1852640, "OUTPUT TRIGGER PERIOD[1]"=1852896, "OUTPUT TRIGGER PERIOD[2]"=1853152, "OUTPUT TRIGGER KIND[0]"=1852656, "OUTPUT TRIGGER KIND[1]"=1852912, "OUTPUT TRIGGER KIND[2]"=1853168, "OUTPUT TRIGGER BASE SENSOR[0]"=1852672, "OUTPUT TRIGGER BASE SENSOR[1]"=1852928, "OUTPUT TRIGGER BASE SENSOR[2]"=1853184, "OUTPUT TRIGGER PRE HSYNC COUNT"=1852704] ("Parameter")
            w537 = u32 1 items=["FORWARD"=1, "BACKWARD"=2] ("Readout Direction")
            w541 = u32 4212128 items=["SENSOR MODE"=4212128, "CCD MODE"=4212384, "READOUT MODE"=4211872, "ACTIVE VIEW INDEX"=4343136, "BITS PER CHANNEL"=4342976, "IMAGE PIXEL TYPE"=4343296, "BINNING"=4215968, "EXPOSURE TIME"=2049184, "CONTRAST GAIN"=3163312, "CONTRAST OFFSET"=3163328, "LIGHT MODE"=2114720, "SENSITIVITY"=2114992, "PHOTON IMAGING MODE"=2115200, "HIGH DYNAMIC RANGE MODE"=3163360, "WHITE BALANCE"=3163568, "TEMPERATURE"=2115232, "TEMPERATURE TARGET"=2115264, "SENSOR COOLER FAN"=2115296, "LINEBUNDLE HEIGHT"=4212192, "MECHANICAL SHUTTER"=2115488, "BACK FOCUS POSITION"=8422304, "TRIGGER CONNECTOR"=1066432, "TRIGGER SOURCE"=1066144, "OUTPUT TRIGGER SOURCE"=1852576, "TRIGGER GLOBAL EXPOSURE"=2049680, "FIRST TRIGGER BEHAVIOR"=2049696, "CHANNEL SYNC"=1852352, "READOUT DIRECTION"=4211904, "PRE HSYNC COUNT"=1852704, "INTERNAL LINE SPEED"=4191408, "INTERNAL LINE INTERVAL"=4191424] ("Parameter")
            w540 = u32 4211904 items=["SENSOR MODE"=4212128, "CCD MODE"=4212384, "READOUT MODE"=4211872, "ACTIVE VIEW INDEX"=4343136, "BITS PER CHANNEL"=4342976, "IMAGE PIXEL TYPE"=4343296, "BINNING"=4215968, "EXPOSURE TIME"=2049184, "CONTRAST GAIN"=3163312, "CONTRAST OFFSET"=3163328, "LIGHT MODE"=2114720, "SENSITIVITY"=2114992, "PHOTON IMAGING MODE"=2115200, "HIGH DYNAMIC RANGE MODE"=3163360, "WHITE BALANCE"=3163568, "TEMPERATURE"=2115232, "TEMPERATURE TARGET"=2115264, "SENSOR COOLER FAN"=2115296, "LINEBUNDLE HEIGHT"=4212192, "MECHANICAL SHUTTER"=2115488, "BACK FOCUS POSITION"=8422304, "TRIGGER CONNECTOR"=1066432, "TRIGGER SOURCE"=1066144, "OUTPUT TRIGGER SOURCE"=1852576, "TRIGGER GLOBAL EXPOSURE"=2049680, "FIRST TRIGGER BEHAVIOR"=2049696, "CHANNEL SYNC"=1852352, "READOUT DIRECTION"=4211904, "PRE HSYNC COUNT"=1852704, "INTERNAL LINE SPEED"=4191408, "INTERNAL LINE INTERVAL"=4191424] ("Parameter")
            n197 = Bundle("Input Trigger Mode"=w519, "Input Trigger Polarity"=w520, "Times"=u32 1, "Delay"=0.0) -> (w516:T13)  [unwired: 1 in]
            n198 = call <userlib>:"tm_setinputtrigger_40.vi"("Parameters"=w516, "Handle in"=w534) -> ("error out"=w514:errorcluster, "Handle out"=w515:u32)  [unwired: 8 in]
            n199 = Bundle("Output Trigger Period"=0.001, "Delay"=0.0, "Source"=w511) -> (w508:T14)  [unwired: 1 in]
            n200 = Bundle("Output Trigger Mode"=w512, "Output Trigger Polarity"=w513) -> (w507:T15)  [unwired: 1 in]
            n201 = call <userlib>:"tm_setoutputtrigger_40.vi"("Port"=1, "error in (no error)"=w514, "Programmable Options"=w508, "Type"=w507, "Handle in"=w515) -> ("error out"=w538:errorcluster, "Handle out"=w539:u32)  [unwired: 5 in]
            n202 = Bundle By Name(cluster=w545, "Received?"=TRUE ("Running?"), "Camera Actions"=Orca_Flash_Actions."Idle") -> (w544:T6)
            n203 = call <userlib>:"tm_setparameter_40.vi"("error in (no error)"=w538, "Value in"=12.0, "Parameter"=w541, "Handle in"=w539) -> ("error out"=w543:errorcluster, "Handle out"=w542:u32)  [unwired: 6 in]
            n204 = To Double Precision Float(number=w537) -> (double precision float=w536:dbl)
            n205 = call <userlib>:"tm_setparameter_40.vi"("error in (no error)"=w543, "Value in"=w536, "Parameter"=w540, "Handle in"=w542) -> ("error out"=w532:errorcluster, "Handle out"=w533:u32)  [unwired: 6 in]
            n206 = call <userlib>:"tm_setparameter_40.vi"("error in (no error)"=w532, "Value in"="Internal Line Interval Setpoint", "Parameter"=w527, "Handle in"=w533) -> ("error out"=w530:errorcluster, "Handle out"=w531:u32)  [unwired: 6 in]
            n207 = call <userlib>:"tm_getparameter_40.vi"("error in (no error)"=w530, "Parameter"=w527, "Handle in"=w531) -> ("error out"=w528:errorcluster, "Value out"=w525:dbl, "Handle out"=w529:u32)  [unwired: 6 in]
            n208 = Multiply(x=w525, y="Number of lines") -> (x*y=w524:dbl)
            n209 = call <userlib>:"tm_setparameter_40.vi"("error in (no error)"=w528, "Value in"=w524, "Parameter"=w521, "Handle in"=w529) -> ("error out"=w522:errorcluster)  [unwired: 6 in, 1 out]
          }
          frame "Area Mode" {
            w553 = u32 2049184 items=["SENSOR MODE"=4212128, "READOUT SPEED"=4211872, "READOUT DIRECTION"=4211904, "TRIGGER GLOBAL EXPOSURE"=2049680, "TRIGGER DELAY"=1066480, "INTERNAL TRIGGER HANDLING"=1066496, "SYNC READOUT SYSTEM BLANK"=1066528, "SENSOR TEMPERATURE"=2115232, "SENSOR COOLER STATUS"=2115280, "EXPOSURE TIME"=2049184, "DEFECT CORRECT MODE"=4670368, "BINNING"=4215968, "INTERNAL LINE SPEED"=4226000, "INTERNAL LINE INTERVAL"=4226016, "NUMBER OF OUTPUT TRIGGER CONNECTOR"=1852320, "OUTPUT TRIGGER SOURCE[0]"=1852576, "OUTPUT TRIGGER SOURCE[1]"=1852832, "OUTPUT TRIGGER SOURCE[2]"=1853088, "OUTPUT TRIGGER POLARITY[0]"=1852592, "OUTPUT TRIGGER POLARITY[1]"=1852848, "OUTPUT TRIGGER POLARITY[2]"=1853104, "OUTPUT TRIGGER ACTIVE[0]"=1852608, "OUTPUT TRIGGER ACTIVE[1]"=1852864, "OUTPUT TRIGGER ACTIVE[2]"=1853120, "OUTPUT TRIGGER DELAY[0]"=1852624, "OUTPUT TRIGGER DELAY[1]"=1852880, "OUTPUT TRIGGER DELAY[2]"=1853136, "OUTPUT TRIGGER PERIOD[0]"=1852640, "OUTPUT TRIGGER PERIOD[1]"=1852896, "OUTPUT TRIGGER PERIOD[2]"=1853152, "OUTPUT TRIGGER KIND[0]"=1852656, "OUTPUT TRIGGER KIND[1]"=1852912, "OUTPUT TRIGGER KIND[2]"=1853168, "OUTPUT TRIGGER BASE SENSOR[0]"=1852672, "OUTPUT TRIGGER BASE SENSOR[1]"=1852928, "OUTPUT TRIGGER BASE SENSOR[2]"=1853184, "OUTPUT TRIGGER PRE HSYNC COUNT"=1852704] ("Parameter")
            w554 = u32 2 items=["NEGATIVE"=1, "POSITIVE"=2] ("Input Trigger Polarity")
            w567 = u32 1 items=["INTERNAL"=1, "EXTERNAL EDGE"=2, "EXTERNAL LEVEL"=4, "SOFTWARE"=32, "FAST REPETITION"=64, "TDI"=128, "START"=512, "SYNC READOUT"=1024] ("Input Trigger Mode")
            w563 = u32 4212128 items=["SENSOR MODE"=4212128, "CCD MODE"=4212384, "READOUT MODE"=4211872, "ACTIVE VIEW INDEX"=4343136, "BITS PER CHANNEL"=4342976, "IMAGE PIXEL TYPE"=4343296, "BINNING"=4215968, "EXPOSURE TIME"=2049184, "CONTRAST GAIN"=3163312, "CONTRAST OFFSET"=3163328, "LIGHT MODE"=2114720, "SENSITIVITY"=2114992, "PHOTON IMAGING MODE"=2115200, "HIGH DYNAMIC RANGE MODE"=3163360, "WHITE BALANCE"=3163568, "TEMPERATURE"=2115232, "TEMPERATURE TARGET"=2115264, "SENSOR COOLER FAN"=2115296, "LINEBUNDLE HEIGHT"=4212192, "MECHANICAL SHUTTER"=2115488, "BACK FOCUS POSITION"=8422304, "TRIGGER CONNECTOR"=1066432, "TRIGGER SOURCE"=1066144, "OUTPUT TRIGGER SOURCE"=1852576, "TRIGGER GLOBAL EXPOSURE"=2049680, "FIRST TRIGGER BEHAVIOR"=2049696, "CHANNEL SYNC"=1852352, "READOUT DIRECTION"=4211904, "PRE HSYNC COUNT"=1852704, "INTERNAL LINE SPEED"=4191408, "INTERNAL LINE INTERVAL"=4191424] ("Parameter")
            n210 = Bundle("Input Trigger Mode"=w567, "Input Trigger Polarity"=w554, "Times"=u32 1, "Delay"=0.0) -> (w564:T13)  [unwired: 1 in]
            n211 = call <userlib>:"tm_setinputtrigger_40.vi"("Parameters"=w564, "Handle in"=w559) -> ("error out"=w561:errorcluster, "Handle out"=w562:u32)  [unwired: 8 in]
            n212 = Bundle By Name(cluster=w556, "Received?"=TRUE ("Running?"), "Camera Actions"=Orca_Flash_Actions."Idle") -> (w555:T6)
            n213 = call <userlib>:"tm_setparameter_40.vi"("error in (no error)"=w561, "Value in"=1.0, "Parameter"=w563, "Handle in"=w562) -> ("error out"=w550:errorcluster, "Handle out"=w551:u32)  [unwired: 6 in]
            n214 = call <userlib>:"tm_setparameter_40.vi"("error in (no error)"=w550, "Value in"=0.1, "Parameter"=w553, "Handle in"=w551) -> ("error out"=w549:errorcluster)  [unwired: 6 in, 1 out]
          }
          frame "Preview" {
            w580 = u32 2049184 items=["SENSOR MODE"=4212128, "READOUT SPEED"=4211872, "READOUT DIRECTION"=4211904, "TRIGGER GLOBAL EXPOSURE"=2049680, "TRIGGER DELAY"=1066480, "INTERNAL TRIGGER HANDLING"=1066496, "SENSOR TEMPERATURE"=2115232, "SENSOR COOLER STATUS"=2115280, "EXPOSURE TIME"=2049184, "DEFECT CORRECT MODE"=4670368, "HOT PIXEL CORRECT LEVEL"=4670400, "BINNING"=4215968, "TIMING READOUT TIME"=4223904, "INTERNAL FRAME RATE"=4225952, "INTERNAL FRAME INTERVAL"=4225968, "INTERNAL LINE SPEED"=4226000, "INTERNAL LINE INTERVAL"=4226016, "IMAGE WIDTH"=4343200, "IMAGE HEIGHT"=4343216, "IMAGE ROWBYTES"=4343232, "IMAGE FRAMEBYTES"=4343248, "IMAGE PIXEL TYPE"=4343296, "NUMBER OF OUTPUT TRIGGER CONNECTOR"=1852320, "OUTPUT TRIGGER SOURCE[0]"=1852576, "OUTPUT TRIGGER SOURCE[1]"=1852832, "OUTPUT TRIGGER SOURCE[2]"=1853088, "OUTPUT TRIGGER POLARITY[0]"=1852592, "OUTPUT TRIGGER POLARITY[1]"=1852848, "OUTPUT TRIGGER POLARITY[2]"=1853104, "OUTPUT TRIGGER ACTIVE[0]"=1852608, "OUTPUT TRIGGER ACTIVE[1]"=1852864, "OUTPUT TRIGGER ACTIVE[2]"=1853120, "OUTPUT TRIGGER DELAY[0]"=1852624, "OUTPUT TRIGGER DELAY[1]"=1852880, "OUTPUT TRIGGER DELAY[2]"=1853136, "OUTPUT TRIGGER PERIOD[0]"=1852640, "OUTPUT TRIGGER PERIOD[1]"=1852896, "OUTPUT TRIGGER PERIOD[2]"=1853152, "OUTPUT TRIGGER KIND[0]"=1852656, "OUTPUT TRIGGER KIND[1]"=1852912, "OUTPUT TRIGGER KIND[2]"=1853168, "OUTPUT TRIGGER BASE SENSOR[0]"=1852672, "OUTPUT TRIGGER BASE SENSOR[1]"=1852928, "OUTPUT TRIGGER BASE SENSOR[2]"=1853184, "OUTPUT TRIGGER PRE HSYNC COUNT"=1852704] ("Parameter")
            w587 = TRUE ("Running?")
            w598 = 1 items=["Snap", "Sequence"] ("Capture mode")
            n215 = Bundle By Name(cluster=w594, "Running?"=w587, "Received?"=w587) -> (w593:T6)
            n216 = call <userlib>:"tm_getparameter_40.vi"("Parameter"=w580, "Handle in"=w581) -> ("error out"=w575:errorcluster, "Value out"=w578:dbl, "Handle out"=w576:u32)  [unwired: 7 in]
            n217 = Send Notification(notification=w593, notifier=w599) -> (notifier out=w596:refnum<notifier>)  [unwired: 1 in, 1 out]
            n218 = Multiply(x=w578, y=5000.0) -> (x*y=w577:dbl)
            n219 = To Long Integer(number=w577) -> (32bit integer=w569:i32)
            n220 = call <userlib>:"tm_preparecapture_40.vi"("error in (no error)"=w575, "Capture mode"=w598, "Handle in"=w576) -> ("error out"=w582:errorcluster, "Handle out"=w583:u32)  [unwired: 5 in, 2 out]
            n221 = call <userlib>:"tm_startcapture_40.vi"("error in (no error)"=w582, "Handle in"=w583) -> ("error out"=w572:errorcluster, "Handle out"=w574:u32)  [unwired: 8 in]
            n222 = call <userlib>:"tm_waitnextframe_40.vi"("error in (no error)"=w572, "Timeout"=5000, "Handle in"=w574) -> ("error out"=w571:errorcluster, "Handle out"=w573:u32)  [unwired: 5 in, 2 out]
            n223 = while {
              tunnel: w596 -> [w609]
              tunnel: [w608] -> w595
              tunnel: w586 -> [w606]
              tunnel: [w605] -> w592
              tunnel: w573 -> [w610]
              tunnel: [w601] -> w597
              tunnel: w571 -> [w604]
              tunnel: w569 -> [w600]
              i -> [w607]
              stop <- w602 stop-if-true
              n224 = Get Notifier Status(notifier=w609) -> (notifier out=w608:refnum<notifier>, current notification=w605:T6)  [unwired: 1 in, 3 out]
              n225 = Unbundle By Name(w605) -> ("Running?"=w603:bool)
              n226 = case shown="True" w603 {
                tunnel: w610 -> [w611 w627]
                tunnel: w606 -> [_ w625]
                tunnel: w604 -> [_ w621]
                tunnel: [TRUE ("status") w618] -> w602
                tunnel: [w611 w617] -> w601
                tunnel: w600 -> [_ w613]
                frame False {
                }
                frame True {
                  n227 = call <userlib>:"tm_waitnextframe_40.vi"("error in (no error)"=w621, "Timeout"=w613, "Handle in"=w627) -> ("error out"=w615:errorcluster, "Frame Count"=w614:i32, "Frame Index"=w624:i32, "Handle out"=w626:u32)  [unwired: 5 in]
                  "Acquisition Frame" <- w614
                  n228 = call <userlib>:"tm_getframe16_40.vi"("error in (no error)"=w615, "Frame Index"=w624, "Handle in"=w626) -> ("error out"=w622:errorcluster, "Data"=w623:u16[][], "Handle out"=w617:u32)  [unwired: 5 in, 1 out]
                  n229 = call "IMAQ ArrayToImage"("Image Pixels (U16)"=w623, "error in (no error)"=w622, "Image"=w625) -> ("error out"=w619:errorcluster, "Image Out"=w620:T8)  [unwired: 7 in]
                  n230 = call "Generic Camera Update Frame Number.vi"("Ref In"=w620, "Frame Number"=w614, "Error In"=w619) -> ("Error Out"=w616:errorcluster)  [unwired: 11 in, 1 out]
                  n231 = Unbundle By Name(w616) -> ("status"=w618:bool)
                }
              }
              "Acquisition Loop" <- w607
            }
            n232 = call <userlib>:"tm_stopcapture_40.vi"("Handle in"=w597) -> ("error out"=w584:errorcluster, "Handle out"=w585:u32)  [unwired: 9 in]
            n233 = Bundle By Name(cluster=w592, "Running?"=FALSE, "Camera Actions"=Orca_Flash_Actions."Idle") -> (w590:T6)
            n234 = call <userlib>:"tm_unpreparecapture_40.vi"("error in (no error)"=w584, "Handle in"=w585) -> ("error out"=w589:errorcluster)  [unwired: 8 in, 1 out]
          }
          frame "Record" {
            w641 = u32 2049184 items=["SENSOR MODE"=4212128, "READOUT SPEED"=4211872, "READOUT DIRECTION"=4211904, "TRIGGER GLOBAL EXPOSURE"=2049680, "TRIGGER DELAY"=1066480, "INTERNAL TRIGGER HANDLING"=1066496, "SENSOR TEMPERATURE"=2115232, "SENSOR COOLER STATUS"=2115280, "EXPOSURE TIME"=2049184, "DEFECT CORRECT MODE"=4670368, "HOT PIXEL CORRECT LEVEL"=4670400, "BINNING"=4215968, "TIMING READOUT TIME"=4223904, "INTERNAL FRAME RATE"=4225952, "INTERNAL FRAME INTERVAL"=4225968, "INTERNAL LINE SPEED"=4226000, "INTERNAL LINE INTERVAL"=4226016, "IMAGE WIDTH"=4343200, "IMAGE HEIGHT"=4343216, "IMAGE ROWBYTES"=4343232, "IMAGE FRAMEBYTES"=4343248, "IMAGE PIXEL TYPE"=4343296, "NUMBER OF OUTPUT TRIGGER CONNECTOR"=1852320, "OUTPUT TRIGGER SOURCE[0]"=1852576, "OUTPUT TRIGGER SOURCE[1]"=1852832, "OUTPUT TRIGGER SOURCE[2]"=1853088, "OUTPUT TRIGGER POLARITY[0]"=1852592, "OUTPUT TRIGGER POLARITY[1]"=1852848, "OUTPUT TRIGGER POLARITY[2]"=1853104, "OUTPUT TRIGGER ACTIVE[0]"=1852608, "OUTPUT TRIGGER ACTIVE[1]"=1852864, "OUTPUT TRIGGER ACTIVE[2]"=1853120, "OUTPUT TRIGGER DELAY[0]"=1852624, "OUTPUT TRIGGER DELAY[1]"=1852880, "OUTPUT TRIGGER DELAY[2]"=1853136, "OUTPUT TRIGGER PERIOD[0]"=1852640, "OUTPUT TRIGGER PERIOD[1]"=1852896, "OUTPUT TRIGGER PERIOD[2]"=1853152, "OUTPUT TRIGGER KIND[0]"=1852656, "OUTPUT TRIGGER KIND[1]"=1852912, "OUTPUT TRIGGER KIND[2]"=1853168, "OUTPUT TRIGGER BASE SENSOR[0]"=1852672, "OUTPUT TRIGGER BASE SENSOR[1]"=1852928, "OUTPUT TRIGGER BASE SENSOR[2]"=1853184, "OUTPUT TRIGGER PRE HSYNC COUNT"=1852704] ("Parameter")
            w647 = TRUE ("Running?")
            w664 = 1 items=["Snap", "Sequence"] ("Capture mode")
            # "First frame takes extra long\nfor capture."
            n235 = Bundle By Name(cluster=w658, "Running?"=w647, "Received?"=w647) -> (w657:T6)
            n236 = Unbundle By Name(w658) -> ("Save Path"=w645:path, "# of frames"=w643:u32)
            n237 = call <userlib>:"tm_getparameter_40.vi"("Parameter"=w641, "Handle in"=w637) -> ("error out"=w636:errorcluster, "Value out"=w639:dbl, "Handle out"=w635:u32)  [unwired: 7 in]
            n238 = Send Notification(notification=w657, notifier=w667) -> (notifier out=w660:refnum<notifier>)  [unwired: 1 in, 1 out]
            n239 = Multiply(x=w639, y=2000.0) -> (x*y=w638:dbl)
            n240 = To Long Integer(number=w638) -> (32bit integer=w628:i32)
            n241 = call "Orca Flash Sort Filenames.vi"("Requested File Path"=w645) -> ("Resulting File Path"=w644:path)  [unwired: 14 in]
            n242 = call <userlib>:"tm_preparecapture_40.vi"("error in (no error)"=w636, "Capture mode"=w664, "Handle in"=w635) -> ("error out"=w666:errorcluster, "Handle out"=w665:u32)  [unwired: 5 in, 2 out]
            n243 = To Long Integer(number=w643) -> (32bit integer=w642:i32)
            n244 = call <userlib>:"tm_startrecorder_40.vi"("error in (no error)"=w666, "frames"=w642, "File"=w644, "Handle in"=w665) -> ("error out"=w652:errorcluster, "Handle out"=w653:u32)  [unwired: 6 in]
            n245 = call <userlib>:"tm_startcapture_40.vi"("error in (no error)"=w652, "Handle in"=w653) -> ("error out"=w632:errorcluster, "Handle out"=w634:u32)  [unwired: 8 in]
            n246 = call <userlib>:"tm_waitnextframe_40.vi"("error in (no error)"=w632, "Timeout"=5000, "Handle in"=w634) -> ("error out"=w631:errorcluster, "Handle out"=w633:u32)  [unwired: 5 in, 2 out]
            n247 = while {
              tunnel: w660 -> [w678]
              tunnel: [w677] -> w659
              tunnel: w646 -> [w676]
              tunnel: [w675] -> w656
              tunnel: w631 -> [w679]
              tunnel: w633 -> [w680]
              tunnel: [w674] -> w663
              tunnel: w642 -> [w672]
              tunnel: w628 -> [w669]
              tunnel: [FALSE] -> w629
              i -> [w673]
              stop <- w670 stop-if-true
              n248 = Get Notifier Status(notifier=w678) -> (notifier out=w677:refnum<notifier>, current notification=w675:T6)  [unwired: 1 in, 3 out]
              n249 = Unbundle By Name(w675) -> ("Running?"=w671:bool)
              n250 = local write "Acquisition Loop"(w673) -> ()
              n251 = case shown="True" w671 {
                tunnel: w680 -> [w682 w700]
                tunnel: w679 -> [_ w699]
                tunnel: w676 -> [_ w697]
                tunnel: [w682 w696] -> w674
                tunnel: w672 -> [_ w691]
                tunnel: [TRUE w684] -> w670
                tunnel: w669 -> [_ w683]
                frame False {
                }
                frame True {
                  n252 = call <userlib>:"tm_waitnextframe_40.vi"("error in (no error)"=w699, "Timeout"=w683, "Handle in"=w700) -> ("error out"=w694:errorcluster, "Frame Count"=w685:i32, "Frame Index"=w695:i32, "Handle out"=w698:u32)  [unwired: 5 in]
                  n253 = Greater Or Equal?(x=w685, y=w691) -> (x >= y?=w688:bool)
                  n254 = call <userlib>:"tm_getframe16_40.vi"("error in (no error)"=w694, "Frame Index"=w695, "Handle in"=w698) -> ("error out"=w692:errorcluster, "Data"=w693:u16[][], "Handle out"=w696:u32)  [unwired: 5 in, 1 out]
                  n255 = local write "Acquisition Frame"(w685) -> ()
                  n256 = call "IMAQ ArrayToImage"("Image Pixels (U16)"=w693, "error in (no error)"=w692, "Image"=w697) -> ("error out"=w689:errorcluster, "Image Out"=w690:T8)  [unwired: 7 in]
                  n257 = call "Generic Camera Update Frame Number.vi"("Ref In"=w690, "Frame Number"=w685, "Error In"=w689) -> ("Error Out"=w686:errorcluster)  [unwired: 11 in, 1 out]
                  n258 = Unbundle By Name(w686) -> ("status"=w687:bool)
                  n259 = Or(x=w687, y=w688) -> (x .or. y?=w684:bool)
                }
              }
            }
            n260 = call <userlib>:"tm_stopcapture_40.vi"("Handle in"=w663) -> ("error out"=w651:errorcluster, "Handle out"=w662:u32)  [unwired: 9 in]
            n261 = local write "Record"(w629) -> ()
            n262 = call <userlib>:"tm_stoprecorder_40.vi"("error in (no error)"=w651, "Handle in"=w662) -> ("error out"=w650:errorcluster, "Handle out"=w661:u32)  [unwired: 8 in]
            n263 = Bundle By Name(cluster=w656, "Running?"=FALSE, "Camera Actions"=Orca_Flash_Actions."Idle") -> (w654:T6)
            n264 = call <userlib>:"tm_unpreparecapture_40.vi"("error in (no error)"=w650, "Handle in"=w661) -> ("error out"=w649:errorcluster)  [unwired: 8 in, 1 out]
          }
          frame "Quit" {
            n265 = call <userlib>:"tm_closecamera_40.vi"("Handle in"=w702) -> ("error out"=w704:errorcluster)  [unwired: 10 in]
            n266 = call "IMAQ Dispose"("Image"=w703) -> ()  [unwired: 5 in, 1 out]
            n267 = Bundle By Name(cluster=w706, "Received?"=TRUE ("Running?")) -> (w705:T6)
            n268 = call <userlib>:"tm_deinitialize_40.vi"("error in (no error)"=w704) -> ("error out"=w701:errorcluster)  [unwired: 10 in]
          }
        }
        "Last Error" <- w363
        n269 = Send Notification(notification=w366, notifier=w369) -> (notifier out=w372:refnum<notifier>)  [unwired: 1 in, 1 out]
      }
      n270 = Release Notifier(notifier=w35, force destroy? (F)=TRUE) -> ()  [unwired: 1 in, 3 out]
    }
    frame Error {
      n271 = call <userlib>:"tm_deinitialize_40.vi"("error in (no error)"=w719) -> ("error out"=w711:errorcluster)  [unwired: 10 in]
      n272 = Release Notifier(notifier=w712, force destroy? (F)=TRUE, error in (no error)=w711) -> (error out=w710:errorcluster)  [unwired: 2 out]
      n273 = Unbundle By Name(w710) -> ("source"=w714:string)
      n274 = call <vilib>:"Space Constant.vi"() -> ("String"=w717:string)
      n275 = Concatenate Strings(w709, w717, "Device Error." ("string"), "\r", w714) -> (w718:string)
      n276 = One Button Dialog(message=w718) -> ()  [unwired: 1 in, 1 out]
    }
  }
